vi "OpenWebsite.vi"   [LabVIEW 2022 SP3]
uses:
  <vilib>/Platform/browser.llb/Open URL in Default Browser (string).vi
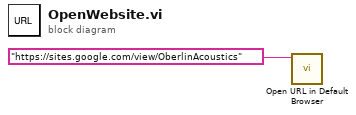
[diagram p0: block diagram]
diagram:
  n1 = call-poly <vilib>:"Open URL in Default Browser.vi"("URL"="https://sites.google.com/view/OberlinAcoustics") -> ()  [unwired: 5 in, 2 out]
